vi "Set window name.vi"(0 "LV Doc.lvclass":refnum<class "LV Doc.lvclass">, 11 "error in (no error)":errorcluster) -> (4 "LV Doc.lvclass":refnum<class "LV Doc.lvclass">, 15 "error out":errorcluster)   [LabVIEW 2016, in "LV Doc.lvclass"]
doc: "Store Window FP title."
uses:
  LV Doc.lvclass
  C:/Users/namratha.balakrishna/Desktop/source code/MDI/D/MDI Project/source code/Document/Document.lvclass
  LV Doc.lvclass/LV Doc.ctl
  Document.lvclass/Document.ctl
  Document.lvclass
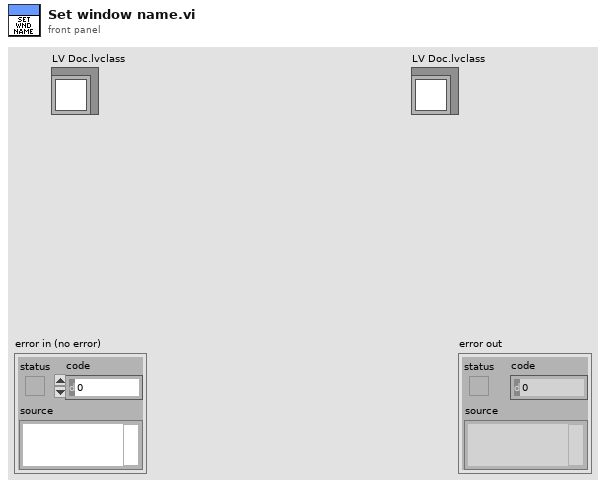
[diagram p1: front panel]
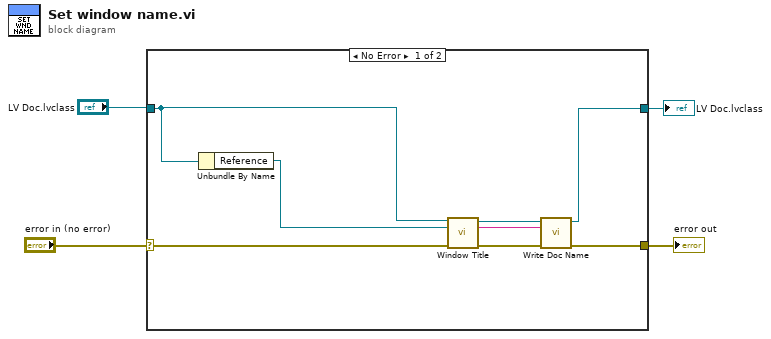
[diagram p0: block diagram]
diagram:
  n1 = case shown="No Error" "error in (no error)" {
    selector: "error in (no error)" -> [w12 w14]
    tunnel: [w11 w14] -> w3
    tunnel: [w10 w13] -> w1
    tunnel: "LV Doc.lvclass" -> [w6 w13]
    frame No Error {
      n2 = Unbundle By Name(w6) -> ("Reference"=w9:refnum<vi>)
      n3 = call-dynamic "Window Title.vi"("LV Doc in"=w6, "VI Reference"=w9, "error in (no error)"=w12) -> ("LV Doc out"=w5:refnum<class "LV Doc.lvclass">, "Window Title"=w7:string, "error out"=w8:errorcluster)  [unwired: 10 in]
      n4 = call "Write Doc Name.vi"("error in (no error)"=w8, "Doc Name"=w7, "Document in"=w5) -> ("error out"=w11:errorcluster, "Document out"=w10:refnum<class "LV Doc.lvclass">)  [unwired: 7 in]
    }
    frame Error {
    }
  }
  "error out" <- w3
  "LV Doc.lvclass" <- w1
